vi "Interpolate Base To object.vi"(7 "Table":dbl[][](array[numeric]), 9 "Z":dbl, 10 "Y":dbl, 11 "X":dbl) -> (1 "z":dbl, 2 "y":dbl, 3 "x":dbl, 5 "a":dbl)   [LabVIEW 2013]
panel:
  out "Numeric":i32
  out "Step":dbl
  # "Object X       ObjectY         ObjectZ        ObjectA         BaseX           BaseY           BaseZ          BaseA"
  # "Far Left"
  # "Far Right"
  # "Near Left"
  # "Near Right"
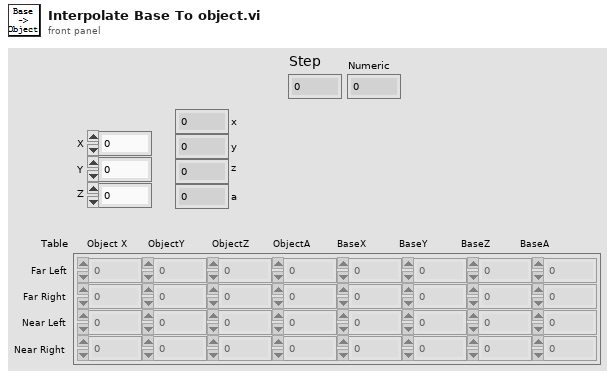
[diagram p1: front panel]
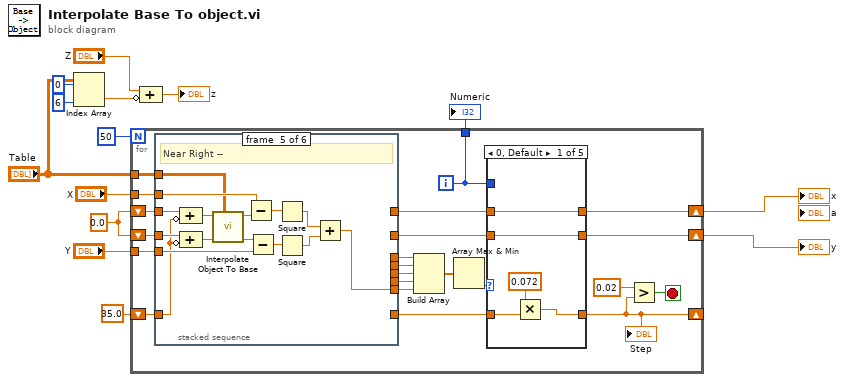
[diagram p0: block diagram]
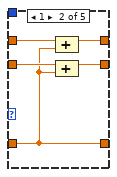
[diagram p2: hidden frame]
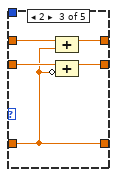
[diagram p3: hidden frame]
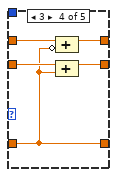
[diagram p4: hidden frame]
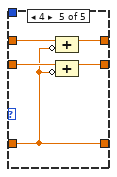
[diagram p5: hidden frame]
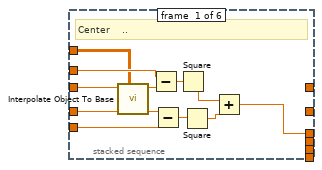
[diagram p6: hidden frame]
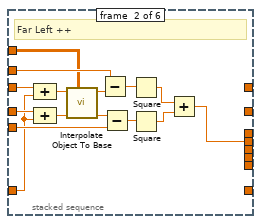
[diagram p7: hidden frame]
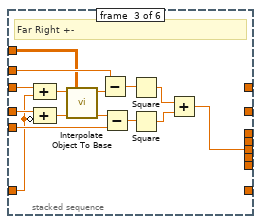
[diagram p8: hidden frame]
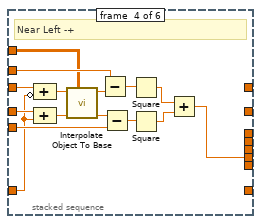
[diagram p9: hidden frame]
diagram:
  w13 = 0.0
  n1 = Index Array(array="Table", index (row)=0 ("disabled index (row)"), index (col)=6 ("disabled index (col)")) -> (element=w3:dbl)
  n2 = for {
    N: 50 -> [_]
    shift-right: [w17] -> w9
    shift-left: w13 -> [w36]
    shift-right: [w22] -> w8
    shift-left: w13 -> [w35]
    shift-right: [w21] -> _
    shift-left: 35.0 -> [w32]
    tunnel: "Y" -> [w34]
    tunnel: "X" -> [w33]
    tunnel: "Table" -> [w18]
    tunnel: [w15] -> w7
    i -> [w15]
    stop <- w20 stop-if-true
    n3 = stacked-sequence {
      tunnel: w36 -> [w73 w80 w95 w110 w125 w136]
      tunnel: w35 -> [w72 w79 w94 w109 w124 w135]
      tunnel: w34 -> [w69 w86 w101 w116 w131 _]
      tunnel: w33 -> [w68 w85 w100 w115 w130 _]
      tunnel: w32 -> [_ w78 w93 w108 w123 w134]
      tunnel: [_ _ _ _ w120 _] -> w31
      tunnel: [_ _ _ w105 _ _] -> w30
      tunnel: [_ _ w90 _ _ _] -> w29
      tunnel: [_ w75 _ _ _ _] -> w28
      tunnel: [w63 _ _ _ _ _] -> w27
      tunnel: [_ _ _ _ _ w136] -> w24
      tunnel: [_ _ _ _ _ w135] -> w23
      tunnel: [_ _ _ _ _ w134] -> w25
      tunnel: w18 -> [w62 w74 w89 w104 w119 _]
      frame #0 {
        # "Center    .."
        n4 = call "Interpolate Object To Base.vi"("Table"=w62, "Y"=w72, "X"=w73) -> ("y"=w70:dbl, "x"=w71:dbl)  [unwired: 5 in, 2 out]
        n5 = Subtract(x=w68, y=w71) -> (x-y=w67:dbl)
        n6 = Subtract(x=w70, y=w69) -> (x-y=w66:dbl)
        n7 = Square(x=w67) -> (x^2=w65:dbl)
        n8 = Square(x=w66) -> (x^2=w64:dbl)
        n9 = Add(x=w65, y=w64) -> (x+y=w63:dbl)
      }
      frame #1 {
        # "Far Left ++"
        n10 = Compound Arithmetic op=ADD(w80, w78) -> (w77:dbl)
        n11 = Compound Arithmetic op=ADD(w79, w78) -> (w76:dbl)
        n12 = call "Interpolate Object To Base.vi"("Table"=w74, "Y"=w76, "X"=w77) -> ("y"=w87:dbl, "x"=w88:dbl)  [unwired: 5 in, 2 out]
        n13 = Subtract(x=w85, y=w88) -> (x-y=w84:dbl)
        n14 = Subtract(x=w87, y=w86) -> (x-y=w83:dbl)
        n15 = Square(x=w84) -> (x^2=w82:dbl)
        n16 = Square(x=w83) -> (x^2=w81:dbl)
        n17 = Add(x=w82, y=w81) -> (x+y=w75:dbl)
      }
      frame #2 {
        # "Far Right +-"
        n18 = Compound Arithmetic op=ADD(w95, w93) -> (w92:dbl)
        n19 = Compound Arithmetic op=ADD(w94, invert w93) -> (w91:dbl)
        n20 = call "Interpolate Object To Base.vi"("Table"=w89, "Y"=w91, "X"=w92) -> ("y"=w102:dbl, "x"=w103:dbl)  [unwired: 5 in, 2 out]
        n21 = Subtract(x=w100, y=w103) -> (x-y=w99:dbl)
        n22 = Subtract(x=w102, y=w101) -> (x-y=w98:dbl)
        n23 = Square(x=w99) -> (x^2=w97:dbl)
        n24 = Square(x=w98) -> (x^2=w96:dbl)
        n25 = Add(x=w97, y=w96) -> (x+y=w90:dbl)
      }
      frame #3 {
        # "Near Left -+"
        n26 = Compound Arithmetic op=ADD(w110, invert w108) -> (w107:dbl)
        n27 = Compound Arithmetic op=ADD(w109, w108) -> (w106:dbl)
        n28 = call "Interpolate Object To Base.vi"("Table"=w104, "Y"=w106, "X"=w107) -> ("y"=w117:dbl, "x"=w118:dbl)  [unwired: 5 in, 2 out]
        n29 = Subtract(x=w115, y=w118) -> (x-y=w114:dbl)
        n30 = Subtract(x=w117, y=w116) -> (x-y=w113:dbl)
        n31 = Square(x=w114) -> (x^2=w112:dbl)
        n32 = Square(x=w113) -> (x^2=w111:dbl)
        n33 = Add(x=w112, y=w111) -> (x+y=w105:dbl)
      }
      frame #4 {
        # "Near Right --"
        n34 = Compound Arithmetic op=ADD(w125, invert w123) -> (w122:dbl)
        n35 = Compound Arithmetic op=ADD(w124, invert w123) -> (w121:dbl)
        n36 = call "Interpolate Object To Base.vi"("Table"=w119, "Y"=w121, "X"=w122) -> ("y"=w132:dbl, "x"=w133:dbl)  [unwired: 5 in, 2 out]
        n37 = Subtract(x=w130, y=w133) -> (x-y=w129:dbl)
        n38 = Subtract(x=w132, y=w131) -> (x-y=w128:dbl)
        n39 = Square(x=w129) -> (x^2=w127:dbl)
        n40 = Square(x=w128) -> (x^2=w126:dbl)
        n41 = Add(x=w127, y=w126) -> (x+y=w120:dbl)
      }
      frame #5 {
      }
    }
    n42 = Build Array(w27, w28, w29, w30, w31) -> (w16:dbl[])
    n43 = Array Max & Min(array=w16) -> (min index (indices)=w26:i32)  [unwired: 3 out]
    n44 = case shown="0, Default" w26 {
      tunnel: w25 -> [w41 w42 w47 w52 w57]
      tunnel: [w40 w42 w47 w52 w57] -> w21
      tunnel: w24 -> [w39 w46 w51 w56 w61]
      tunnel: w23 -> [w38 w45 w50 w55 w60]
      tunnel: [w39 w44 w49 w54 w59] -> w17
      tunnel: [w38 w43 w48 w53 w58] -> w22
      tunnel: w15 -> [_ _ _ _ _]
      frame 0, Default {
        n45 = Multiply(x=0.072 ("x 2"), y=w41) -> (x*y=w40:dbl)
      }
      frame 1 {
        n46 = Compound Arithmetic op=ADD(w46, w42) -> (w44:dbl)
        n47 = Compound Arithmetic op=ADD(w45, w42) -> (w43:dbl)
      }
      frame 2 {
        n48 = Compound Arithmetic op=ADD(w51, w47) -> (w49:dbl)
        n49 = Compound Arithmetic op=ADD(w50, invert w47) -> (w48:dbl)
      }
      frame 3 {
        n50 = Compound Arithmetic op=ADD(w56, invert w52) -> (w54:dbl)
        n51 = Compound Arithmetic op=ADD(w55, w52) -> (w53:dbl)
      }
      frame 4 {
        n52 = Compound Arithmetic op=ADD(w61, invert w57) -> (w59:dbl)
        n53 = Compound Arithmetic op=ADD(w60, invert w57) -> (w58:dbl)
      }
    }
    "Step" <- w21
    n54 = Greater?(x=0.02, y=w21) -> (0:w20:bool)
  }
  "x" <- w9
  "y" <- w8
  "Numeric" <- w7
  n55 = Compound Arithmetic op=ADD("Z", invert w3) -> (→"z":dbl)
